vi "readwordexcels(1).vi"() -> (14 "cases":string[](array[string]))   [LabVIEW 2021]
uses:
  <vilib>/Utility/NIReport.llb/NI_report.lvclass
  <vilib>/Utility/NIReport.llb/Word/NI_Word.lvclass
panel:
  out "x+y":i32
  in  "错误输入（无错误）":errorcluster
  out "Text 2":string
  out "Count 4":i32
  out "Count 3":i32
  out "NestingLevel":i32
  out "Parent":variant
  out "Count":i32
  out "Text":string
  in  "template (empty)":path
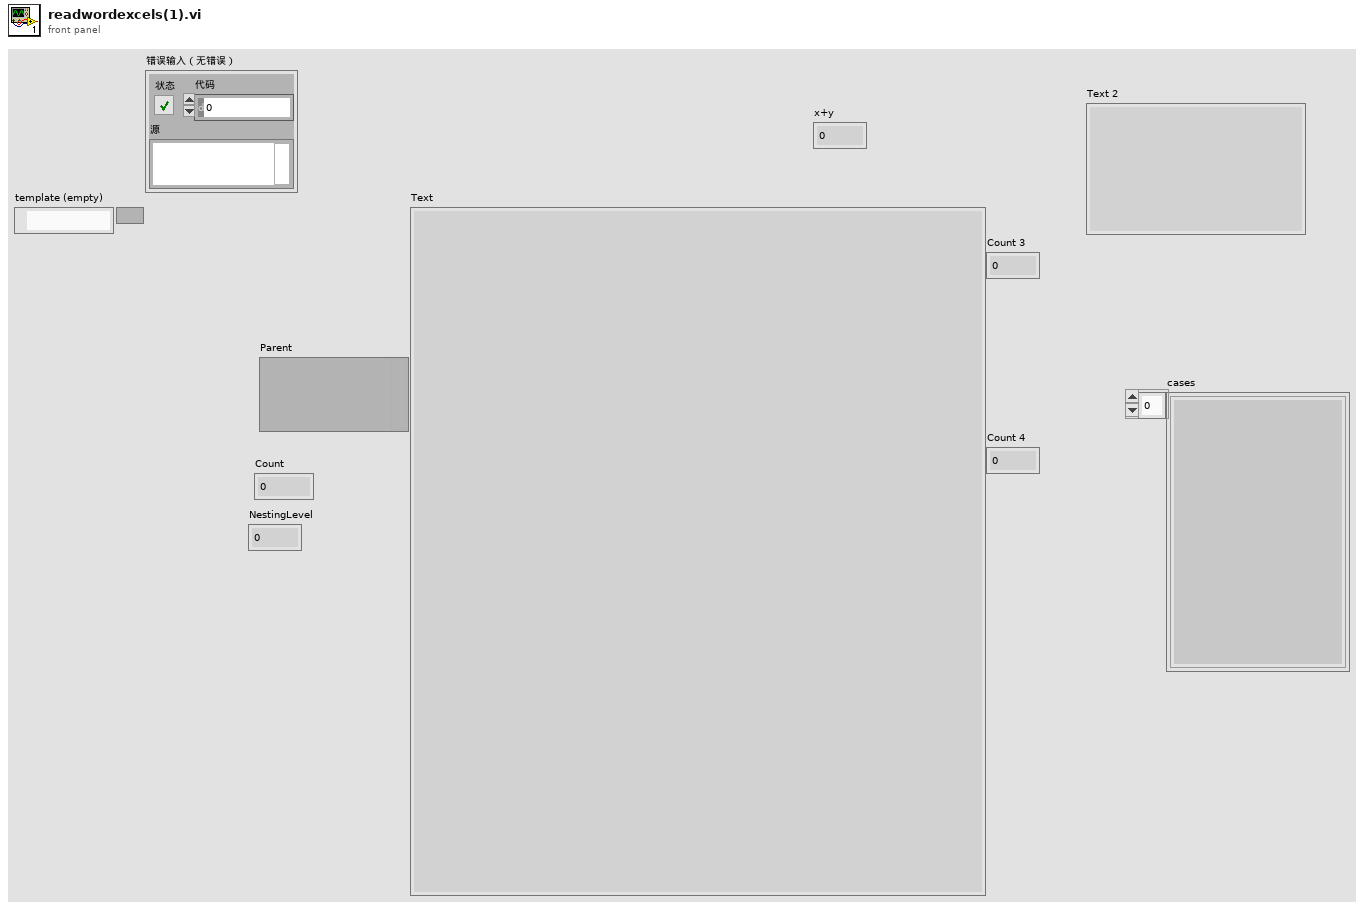
[diagram p1: front panel]
types:
  T1 = enum16{"Standard Report", "HTML", "Word", "Excel"}
  T2 = enum16{"maximized", "minimized", "normal", "no change"}
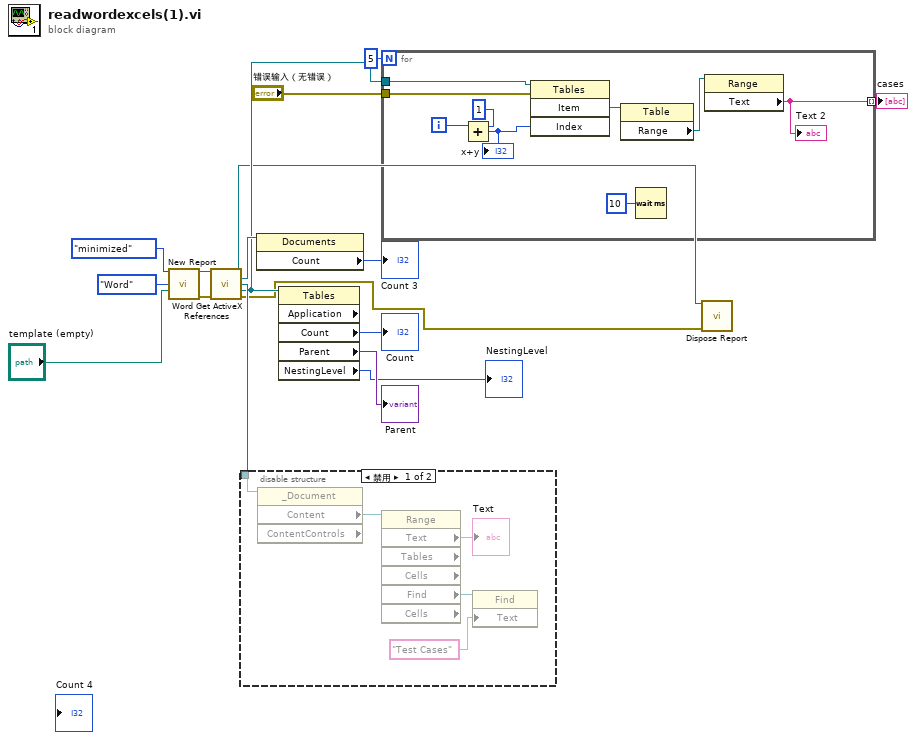
[diagram p0: block diagram]
diagram:
  n1 = call <vilib>:"New Report.vi"("window state (normal)"=T2."minimized", "report type"=T1."Word", "template (empty)"="template (empty)") -> ("report out"=w13:refnum<class "NI_report.lvclass">, "error out"=w15:errorcluster)  [unwired: 11 in]
  n2 = call <vilib>:"Word Get ActiveX References.vi"("report in"=w13, "error in (no error)"=w15) -> ("report out"=w5:refnum<class "NI_report.lvclass">, "Word.Documents"=w10:refnum<k7>, "Word._Document"=w14:refnum<k7>, "Word.Tables"=w6:refnum<k7>, "error out"=w4:errorcluster)  [unwired: 7 in, 2 out]
  n3 = disable-structure shown="禁用" {
    disable-tunnel: w14 -> [w22 _]
    frame Disabled {
      n4 = property class="_Document" props=["Content", "ContentControls"](reference=w22) -> ("Content"=w21:refnum<k7>)  [unwired: 1 in, 3 out]
      n5 = property class="Range" props=["Text", "Tables", "Cells", "Find", "Cells"](reference=w21) -> ("Text"=→"Text":string, "Find"=w19:refnum<k7>)  [unwired: 1 in, 5 out]
      n6 = property class="Find"(reference=w19, "Text"="Test Cases") -> ()  [unwired: 1 in, 2 out]
    }
    frame Enabled {
    }
  }
  n7 = property class="Documents"(reference=w10) -> ("Count"=→"Count 3":i32)  [unwired: 1 in, 2 out]
  n8 = property class="Tables" props=["Application", "Count", "Parent", "NestingLevel"](reference=w6) -> ("Count"=→"Count":i32, "Parent"=→"Parent":variant, "NestingLevel"=→"NestingLevel":i32)  [unwired: 1 in, 3 out]
  n9 = for {
    N: 5 -> [_]
    tunnel: w6 -> [w31]
    tunnel: [w28] -> w8 mode=indexing
    tunnel: "错误输入（无错误）" -> [w24]
    i -> [w27]
    n10 = Add(x=1, y=w27) -> (x+y=w25:i32)
    "x+y" <- w25
    n11 = invoke class="Tables" method="Item"(reference=w31, error in=w24, "Index"=w25) -> ("Item"=w30:refnum<k7>)  [unwired: 1 in, 3 out]
    n12 = property class="Table"(reference=w30) -> ("Range"=w29:refnum<k7>)  [unwired: 1 in, 2 out]
    n13 = Wait (ms)(milliseconds to wait=u32 10 ("等待时间（毫秒）")) -> ()  [unwired: 1 out]
    n14 = property class="Range"(reference=w29) -> ("Text"=w28:string)  [unwired: 1 in, 2 out]
    "Text 2" <- w28
  }
  "cases" <- w8
  n15 = call-dynamic "Dispose Report.vi"("report in"=w5, "error in (no error)"=w4) -> ()  [unwired: 13 in, 1 out]
